vi "Car Entered.vi"(11 "IO":T1) -> (3 "bt_Node out":refnum<class "bt_Node.lvclass">)   [LabVIEW 2021, in "Car Wash Support.lvlib"]
uses:
  Car Wash Support.lvlib
  IO Refs.ctl
  <vilib>/TSA/Event Log/Event_TextLog/Event_TextLog.lvclass
  C:/Program Files (x86)/National Instruments/LabVIEW 2021/vi.lib/TSA/Event Log/abs_EventLog/abs_EventLog.lvclass
  <vilib>/TSA/Abstract Data Classes/Abs_Types/Boolean/Abs_Boolean.lvclass
  C:/Program Files (x86)/National Instruments/LabVIEW 2021/vi.lib/TSA/Abstract Data Classes/Abs_Types/Value/Abs_Value.lvclass
  C:/Program Files (x86)/National Instruments/LabVIEW 2021/vi.lib/TSA/Abstract Data Classes/Abs_Types/Type/Abs_Type.lvclass
  <vilib>/TSA/Abstract Data Classes/Abs_Types/I32 Integer/Abs_I32 Integer.lvclass
  C:/Program Files (x86)/National Instruments/LabVIEW 2021/vi.lib/TSA/Abstract Data Classes/Abs_Types/Numeric/Abs_Numeric.lvclass
  <vilib>/TSA/Abstract Data Classes/Abs_Types/Double Float/Abs_Double Float.lvclass
  Wash Indicators.ctl
  Wash Options.ctl
  Support/Nodes/abs_Node/bt_Node.lvclass
  Support/Nodes/Decorators/Repeater/Support/Finish On - Type.ctl
  Support/Nodes/Leaves/abs_Type Leaf/abs_Type Leaf.lvclass/abs_Type Leaf.ctl
  Support/Nodes/Leaves/abs_Type Leaf/Properties/Write Value Class.vi
  Support/Nodes/Leaves/Test Boolean/Test Abs_Boolean.lvclass
  C:/Users/timst/Documents/Repositories/LV_Behaviour_Tree/Source/Support/Nodes/abs_Node/bt_Node.lvclass
  C:/Users/timst/Documents/Repositories/LV_Behaviour_Tree/Source/Support/Nodes/Leaves/abs_Type Leaf/abs_Type Leaf.lvclass
  Support/Nodes/Leaves/Log/bt_Log.lvclass
  <vilib>/TSA/Abstract Data Classes/Constants/Support/Str/Str.vi
  <vilib>/TSA/Abstract Data Classes/Constants/Support/I32/I32.vi
  Support/Poly/Log/Log_StringClass.vi
  <vilib>/TSA/Abstract Data Classes/Functions/Compare/Support/Equal/I32/Method.vi
  <vilib>/TSA/Abstract Data Classes/Constants/Support/Bool/Bool.vi
  BT.lvlib
  <vilib>/TSA/Abstract Data Classes/Constants/Support/Bool/Const_Bool.lvclass
  <vilib>/TSA/Abstract Data Classes/Constants/Support/Str/Const_Str.lvclass
  Support/Nodes/Decorators/Repeater/bt_Repeater.lvclass
  <vilib>/TSA/Abstract Data Classes/Constants/Support/I32/Const_I32.lvclass
  <vilib>/TSA/Abstract Data Classes/Functions/Compare/Support/Equal/I32/Equal_I32.lvclass
  C:/Program Files (x86)/National Instruments/LabVIEW 2021/vi.lib/TSA/Abstract Data Classes/Abs_Types/Integer/Abs_Integer.lvclass
  C:/Program Files (x86)/National Instruments/LabVIEW 2021/vi.lib/TSA/Abstract Data Classes/Abs_Types/I32 Integer/Abs_I32 Integer.lvclass
  C:/Program Files (x86)/National Instruments/LabVIEW 2021/vi.lib/TSA/Event Log/Event_TextLog/Event_TextLog.lvclass
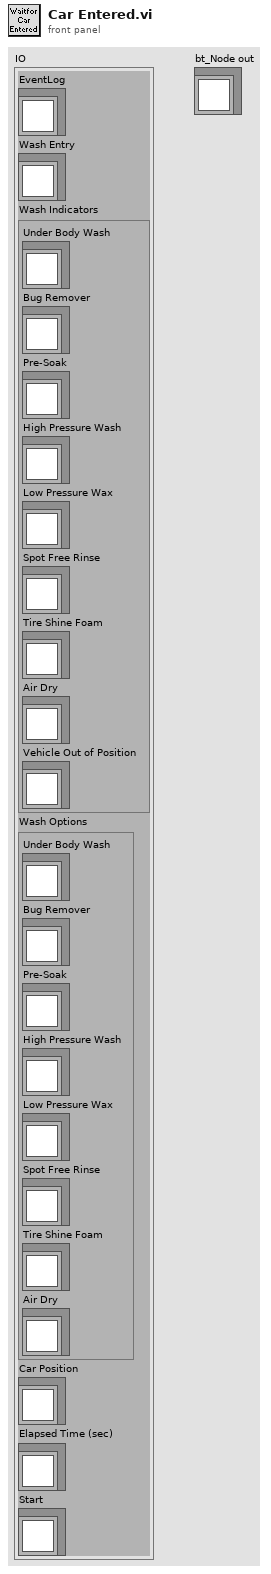
[diagram p1: front panel]
types:
  T1 = typedef "Car Wash Support.lvlib/IO Refs.ctl" = cluster{"EventLog":refnum<class "Event_TextLog.lvclass">, "Wash Entry":refnum<class "Abs_Boolean.lvclass">, "Wash Indicators":T2, "Wash Options":T3, "Car Position":refnum<class "Abs_I32 Integer.lvclass">, "Elapsed Time (sec)":refnum<class "Abs_Double Float.lvclass">, "Start":refnum<class "Abs_Boolean.lvclass">}
  T2 = typedef "Car Wash Support.lvlib/Wash Indicators.ctl" = cluster{"Under Body Wash":refnum<class "Abs_Boolean.lvclass">, "Bug Remover":refnum<class "Abs_Boolean.lvclass">, "Pre-Soak":refnum<class "Abs_Boolean.lvclass">, "High Pressure Wash":refnum<class "Abs_Boolean.lvclass">, "Low Pressure Wax":refnum<class "Abs_Boolean.lvclass">, "Spot Free Rinse":refnum<class "Abs_Boolean.lvclass">, "Tire Shine Foam":refnum<class "Abs_Boolean.lvclass">, "Air Dry":refnum<class "Abs_Boolean.lvclass">, "Vehicle Out of Position":refnum<class "Abs_Boolean.lvclass">}
  T3 = typedef "Car Wash Support.lvlib/Wash Options.ctl" = cluster{"Under Body Wash":refnum<class "Abs_Boolean.lvclass">, "Bug Remover":refnum<class "Abs_Boolean.lvclass">, "Pre-Soak":refnum<class "Abs_Boolean.lvclass">, "High Pressure Wash":refnum<class "Abs_Boolean.lvclass">, "Low Pressure Wax":refnum<class "Abs_Boolean.lvclass">, "Spot Free Rinse":refnum<class "Abs_Boolean.lvclass">, "Tire Shine Foam":refnum<class "Abs_Boolean.lvclass">, "Air Dry":refnum<class "Abs_Boolean.lvclass">}
  T4 = typedef "BT.lvlib/bt_Repeater.lvclass/Finish On - Type.ctl" = enum16{"Success", "Failure", "Never"}
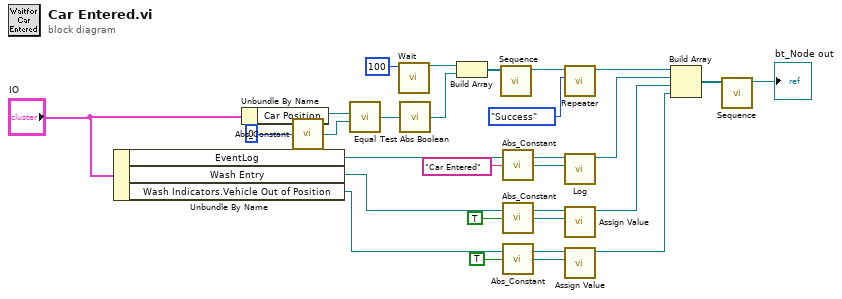
[diagram p0: block diagram]
diagram:
  n1 = Unbundle By Name("IO") -> ("EventLog"=w26:refnum<class "Event_TextLog.lvclass">, "Wash Entry"=w11:refnum<class "Abs_Boolean.lvclass">, "Wash Indicators.Vehicle Out of Position"=w7:refnum<class "Abs_Boolean.lvclass">)
  n2 = Unbundle By Name("IO") -> ("Car Position"=w20:refnum<class "Abs_I32 Integer.lvclass">)
  n3 = call-poly <vilib>:"Abs_Constant.vi"("Value"=0) -> ("Constant"=w23:refnum<class "Abs_I32 Integer.lvclass">)  [unwired: 4 in]
  n4 = call-poly <vilib>:"Equal.vi"("Value B"=w23, "Value A"=w20) -> ("Result"=w21:refnum<class "Abs_Boolean.lvclass">)  [unwired: 4 in]
  n5 = call "Wait.vi"("Time (ms)"=u32 100) -> ("Node Out"=w5:refnum<class "bt_Node.lvclass">)  [unwired: 10 in]
  n6 = call "Test Abs Boolean.vi"("Abs_Boolean.lvclass"=w21) -> ("abs_Node"=w4:refnum<class "bt_Node.lvclass">)  [unwired: 4 in]
  n7 = Build Array(w5, w4) -> (w6:refnum<class "bt_Node.lvclass">[])
  n8 = call "Sequence.vi"("Nodes"=w6) -> ("Node"=w3:refnum<class "bt_Node.lvclass">)  [unwired: 10 in]
  n9 = call-poly <vilib>:"Abs_Constant.vi"("String"="Car Entered") -> ("Abs_String.lvclass"=w15:refnum<class "Abs_String.lvclass">)  [unwired: 4 in]
  n10 = call-poly <vilib>:"Abs_Constant.vi"("Boolean"=TRUE) -> ("Abs_Boolean.lvclass"=w14:refnum<class "Abs_Boolean.lvclass">)  [unwired: 4 in]
  n11 = call-poly <vilib>:"Abs_Constant.vi"("Boolean"=TRUE) -> ("Abs_Boolean.lvclass"=w9:refnum<class "Abs_Boolean.lvclass">)  [unwired: 4 in]
  n12 = call "Repeater.vi"("Finish On"=Finish_On_-_Type."Success", "Node In"=w3) -> ("Node Out"=w1:refnum<class "bt_Node.lvclass">)  [unwired: 9 in]
  n13 = call-poly "Log.vi"("Message"=w15, "EventLog"=w26) -> ("node out"=w16:refnum<class "bt_Log.lvclass">)  [unwired: 9 in]
  n14 = call "Assign Value.vi"("Assigned Value"=w14, "Value"=w11) -> ("Node Out"=w12:refnum<class "bt_Node.lvclass">)  [unwired: 9 in]
  n15 = call "Assign Value.vi"("Assigned Value"=w9, "Value"=w7) -> ("Node Out"=w8:refnum<class "bt_Node.lvclass">)  [unwired: 9 in]
  n16 = Build Array(w1, w16, w12, w8) -> (w18:refnum<class "bt_Node.lvclass">[])
  n17 = call "Sequence.vi"("Nodes"=w18) -> ("Node"=→"bt_Node out":refnum<class "bt_Node.lvclass">)  [unwired: 10 in]
